vi "Agilent PWM Set Remote.vi"(8 "error in (no error)":errorcluster, 11 "VISA Resource Name":refnum<visa-resource-name>) -> (0 "error out":errorcluster, 3 "dup VISA Resource Name":refnum<visa-resource-name>)   [LabVIEW 2011]
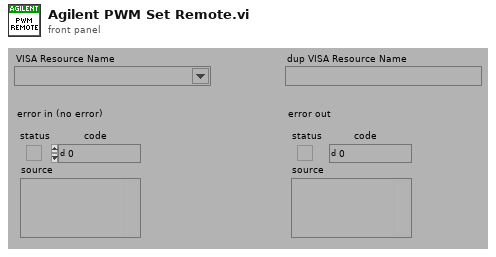
[diagram p1: front panel]
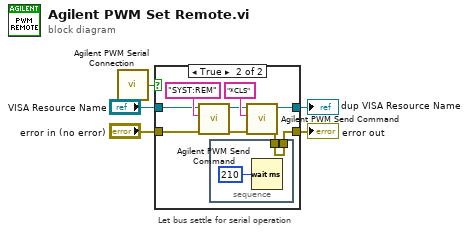
[diagram p0: block diagram]
diagram:
  # "Let bus settle for serial operation"
  n1 = call "Agilent PWM Serial Connection.vi"("VISA Resource Name"="VISA Resource Name") -> ("Serial?"=w2:bool)
  n2 = case shown="True" w2 {
    tunnel: "VISA Resource Name" -> [w7 w14]
    tunnel: "error in (no error)" -> [w6 w13]
    tunnel: [w7 w9] -> w4
    tunnel: [w6 w16] -> w3
    frame False {
    }
    frame True {
      n3 = call "Agilent PWM Send Command.vi"("error in (no error)"=w13, "Command"="SYST:REM", "VISA Resource Name"=w14) -> ("error out"=w11:errorcluster, "dup VISA Resource Name"=w10:refnum<visa-resource-name>)  [unwired: 3 in, 4 out]
      n4 = call "Agilent PWM Send Command.vi"("error in (no error)"=w11, "Command"="*CLS", "VISA Resource Name"=w10) -> ("error out"=w8:errorcluster, "dup VISA Resource Name"=w9:refnum<visa-resource-name>)  [unwired: 3 in, 4 out]
      n5 = stacked-sequence {
        tunnel: w8 -> [w17]
        tunnel: [w17] -> w16
        frame #0 {
          n6 = Wait (ms)(milliseconds to wait=u32 210) -> ()  [unwired: 1 out]
        }
      }
    }
  }
  "dup VISA Resource Name" <- w4
  "error out" <- w3
